vi "Master Configure Clock.vi"(8 "error in":errorcluster, 10 "Clock Source":T2(ring), 11 "Master Ref":T1) -> (0 "error out":errorcluster, 2 "Configuration Error":bool, 3 "Master Ref":T1)   [LabVIEW 2015]
doc: "This VI configures the clock source for the NI 5782. For execution steps, refer to the comments on the block diagram."
uses:
  Controls/FpgaMasterRef Typedef.ctl
  <vilib>/Utility/error.llb/Error Cluster From Error Code.vi
  <vilib>/rvi/errors/niLvFpgaAdjustHostInterfaceError.vi
  <vilib>/rvi/interface/nirviReadWriteControl/nirviReadWriteControl.xnode
  FPGA Bitfiles/LidarMasterV5.2.1.lvbitx
  NiFpgaLv.dll
panel:
  out "PLL Locked 2":bool
  out "ref":i32
  out "PLL Locked":bool
  # "This VI configures the clock source for the NI 5771. For execution steps, refer to the comments on the block diagram."
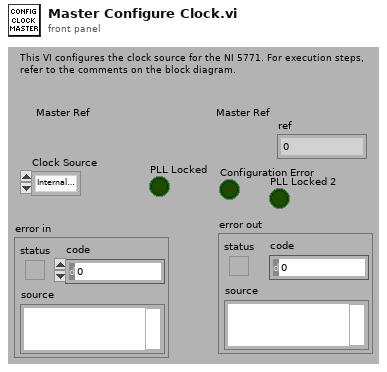
[diagram p1: front panel]
types:
  T1 = typedef "FpgaMasterRef Typedef.ctl" = refnum<k20>
  T2 = enum8{"Internal Clock PLL Off", "Internal Clock PLL On (CLK IN)", "External Clock (CLK IN)", "Internal Clock PLL On (IoModSyncClock)", "Extrernal Clock (IoModSyncClk)"}
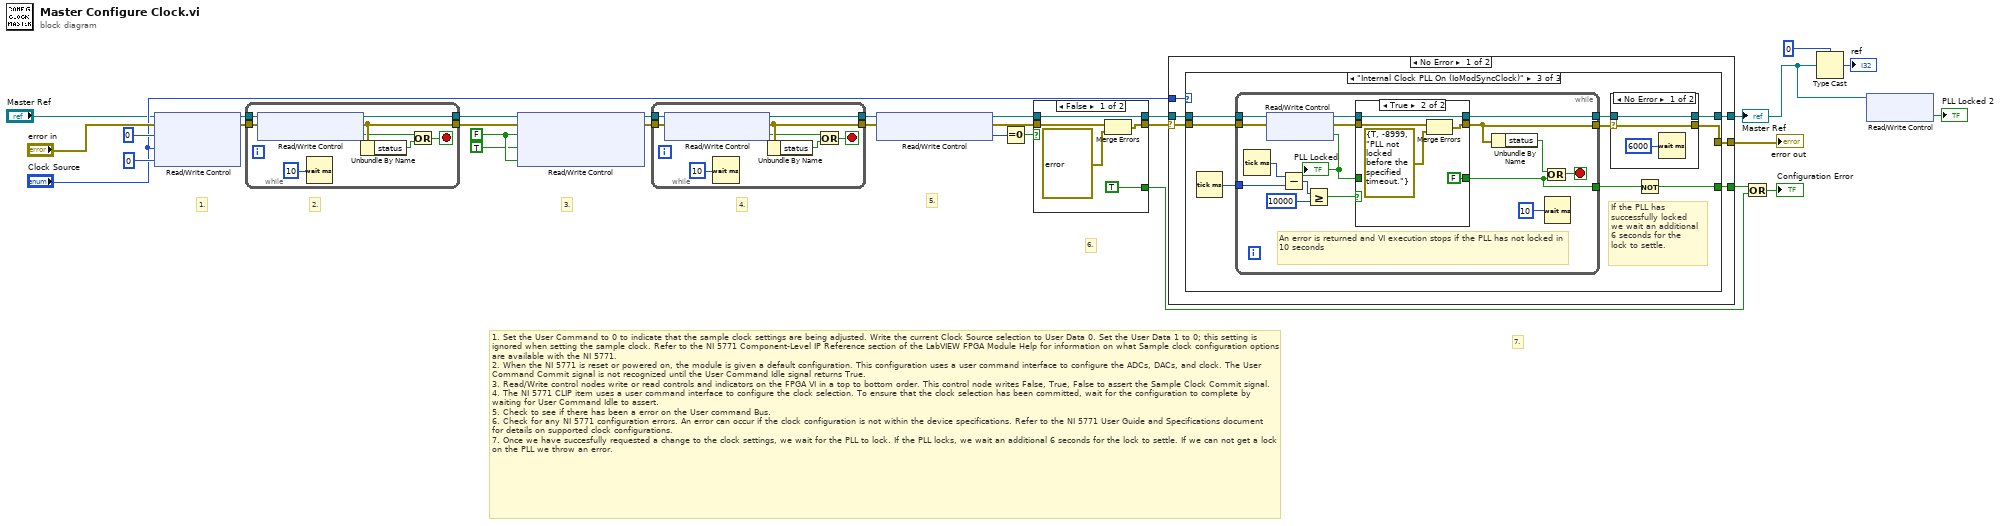
[diagram p0: block diagram]
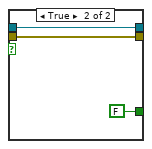
[diagram p2: hidden frame]
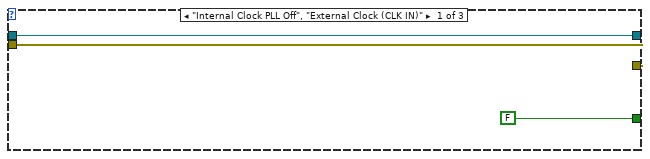
[diagram p3: hidden frame]
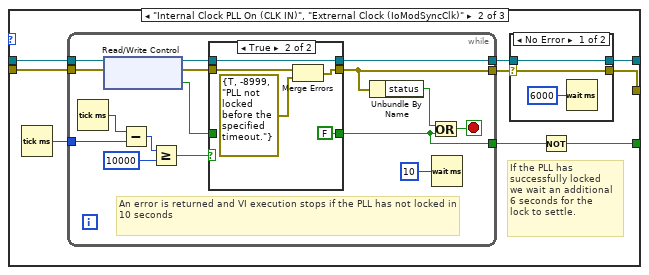
[diagram p4: hidden frame]
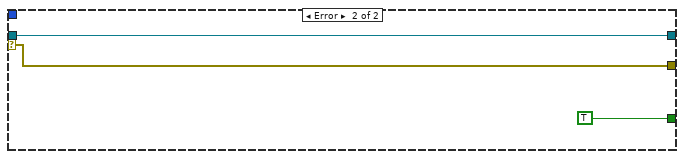
[diagram p9: hidden frame]
diagram:
  w24 = FALSE ("Sample Clock Commit")
  # "6."
  # "5."
  # "7."
  # "1. Set the User Command to 0 to indicate that the sample clock settings are being adjusted. Write the current Clock Source selection to User Data 0. Set the User Data 1 to 0; this setting is ignored when setting the sample clock. Refer to the NI 5771 Component-Level IP Reference section of the LabVIEW FPGA Module Help for information on what Sample clock configuration options are available with the NI 5771.\n2. When the NI 5771 is reset or powered on, the module is given a default configuration. This configuration uses a user command interface to configure the ADCs, DACs, and clock. The User Command Commit signal is not recognized until the User Command Idle signal returns True.\n3. Read/Write control nodes write or read controls and indicators on the FPGA VI in a top to bottom order. This control node writes False, True, False to assert the Sample Clock Commit signal.\n4. The NI 5771 CLIP item uses a user command interface to configure the clock selection. To ensure that the clock selection has been committed, wait for the configuration to complete by waiting for User Command Idle to assert.\n5. Check to see if there has been a error on the User command Bus. \n6. Check for any NI 5771 configuration errors. An error can occur if the clock configuration is not within the device specifications. Refer to the NI 5771 User Guide and Specifications document for details on supported clock configurations.\n7. Once we have succesfully requested a change to the clock settings, we wait for the PLL to lock. If the PLL locks, we wait an additional 6 seconds for the lock to settle. If we can not get a lock on the PLL we throw an error."
  # "4."
  # "3."
  # "2."
  # "1."
  n1 = xnode "Read/Write Control"("FPGA VI Reference In"="Master Ref", "error in"="error in", "User Command"=u8 0, "User Data 0"="Clock Source", "User Data 1"=u8 0) -> ("FPGA VI Reference Out"=w28:T1, "error out"=w27:errorcluster)
  n2 = while {
    tunnel: w28 -> [w33]
    tunnel: w27 -> [w34]
    tunnel: [w31] -> w25
    tunnel: [w32] -> w26
    stop <- w35 stop-if-true
    n3 = xnode "Read/Write Control"("FPGA VI Reference In"=w33, "error in"=w34) -> ("FPGA VI Reference Out"=w32:T1, "error out"=w31:errorcluster, "User Command Idle"=w30:bool)
    n4 = Wait (ms)(milliseconds to wait=u32 10) -> ()  [unwired: 1 out]
    n5 = Unbundle By Name(w31) -> ("status"=w36:bool)
    n6 = Or(x=w30, y=w36) -> (x .or. y?=w35:bool)
  }
  n7 = xnode "Read/Write Control"("FPGA VI Reference In"=w26, "error in"=w25, "User Command Commit"=w24, "User Command Commit"=TRUE ("Sample Clock Commit"), "User Command Commit"=w24) -> ("FPGA VI Reference Out"=w22:T1, "error out"=w21:errorcluster)
  n8 = while {
    tunnel: w22 -> [w41]
    tunnel: w21 -> [w42]
    tunnel: [w39] -> w20
    tunnel: [w40] -> w19
    stop <- w43 stop-if-true
    n9 = xnode "Read/Write Control"("FPGA VI Reference In"=w41, "error in"=w42) -> ("FPGA VI Reference Out"=w40:T1, "error out"=w39:errorcluster, "User Command Idle"=w38:bool)
    n10 = Wait (ms)(milliseconds to wait=u32 10) -> ()  [unwired: 1 out]
    n11 = Unbundle By Name(w39) -> ("status"=w44:bool)
    n12 = Or(x=w38, y=w44) -> (x .or. y?=w43:bool)
  }
  n13 = xnode "Read/Write Control"("FPGA VI Reference In"=w19, "error in"=w20) -> ("FPGA VI Reference Out"=w7:T1, "error out"=w9:errorcluster, "User Command Status"=w8:u8)
  n14 = Equal To 0?(x=w8) -> (x = 0?=w6:bool)
  n15 = case shown="False" w6 {
    tunnel: [w50 w53] -> w15
    tunnel: w9 -> [w49 w53]
    tunnel: [TRUE ("Configured?") FALSE ("Configured?")] -> w10
    tunnel: w7 -> [w46 w51]
    tunnel: [w46 w51] -> w13
    frame False {
      n16 = Merge Errors(w49, errorcluster {"status"=TRUE, "code"=-8998, "source"="IO Module clock not configured correctly. Please ensure that the desired clock meets the required specifications."} ("error in")) -> (w50:errorcluster)
    }
    frame True {
    }
  }
  n17 = case shown="No Error" w15 {
    selector: w15 -> [w57 w140]
    tunnel: "Clock Source" -> [w59 _]
    tunnel: w13 -> [w58 w141]
    tunnel: [w56 w140] -> w14
    tunnel: [w55 w141] -> w2
    tunnel: [w54 TRUE ("Configured?")] -> w12
    frame No Error {
      n18 = case shown="\"Internal Clock PLL On (IoModSyncClock)\"" w59 {
        tunnel: w58 -> [w61 w70 w108]
        tunnel: w57 -> [w62 w69 w107]
        tunnel: [w62 w66 w104] -> w56
        tunnel: [w61 w67 w105] -> w55
        tunnel: [FALSE ("Configured?") w63 w101] -> w54
        frame "Internal Clock PLL Off", "External Clock (CLK IN)" {
        }
        frame "Internal Clock PLL On (CLK IN)", "Extrernal Clock (IoModSyncClk)" {
          # "If the PLL has \nsuccessfully locked \nwe wait an additional\n6 seconds for the \nlock to settle."
          n19 = Tick Count (ms)() -> (millisecond timer value=w71:u32)
          n20 = while {
            tunnel: [w90] -> w68
            tunnel: w70 -> [w87]
            tunnel: w71 -> [w83]
            tunnel: w69 -> [w81]
            tunnel: [w78] -> w65
            tunnel: [w77] -> w64
            stop <- w88 stop-if-true
            # "An error is returned and VI execution stops if the PLL has not locked in 10 seconds"
            n21 = Tick Count (ms)() -> (millisecond timer value=w84:u32)
            n22 = xnode "Read/Write Control"("FPGA VI Reference In"=w87, "error in"=w81) -> ("FPGA VI Reference Out"=w79:T1, "error out"=w85:errorcluster, "PLL Locked"=w86:bool)
            n23 = Subtract(x=w84, y=w83) -> (x-y=w82:u32)
            n24 = Greater Or Equal?(x=w82, y=u32 10000) -> (x >= y?=w91:bool)
            n25 = case shown="True" w91 {
              tunnel: [w95 FALSE ("Configured?")] -> w77
              tunnel: w86 -> [w95 _]
              tunnel: [w94 w99] -> w90
              tunnel: w85 -> [w94 w97]
              tunnel: w79 -> [w93 w96]
              tunnel: [w93 w96] -> w78
              frame False {
              }
              frame True {
                n26 = Merge Errors(w97, errorcluster {"status"=TRUE, "code"=-8999, "source"="PLL not locked before the specified timeout."} ("error in")) -> (w99:errorcluster)
              }
            }
            n27 = Unbundle By Name(w90) -> ("status"=w89:bool)
            n28 = Or(x=w89, y=w77) -> (x .or. y?=w88:bool)
            n29 = Wait (ms)(milliseconds to wait=u32 10) -> ()  [unwired: 1 out]
          }
          n30 = case shown="No Error" w68 {
            selector: w68 -> [w72 w76]
            tunnel: w65 -> [w73 w75]
            tunnel: [w73 w75] -> w67
            tunnel: [w72 w76] -> w66
            frame No Error {
              n31 = Wait (ms)(milliseconds to wait=u32 6000) -> ()  [unwired: 1 out]
            }
            frame Error {
            }
          }
          n32 = Not(x=w64) -> (.not. x?=w63:bool)
        }
        frame "Internal Clock PLL On (IoModSyncClock)" {
          # "If the PLL has \nsuccessfully locked \nwe wait an additional\n6 seconds for the \nlock to settle."
          n33 = Tick Count (ms)() -> (millisecond timer value=w109:u32)
          n34 = while {
            tunnel: [w128] -> w106
            tunnel: w108 -> [w125]
            tunnel: w109 -> [w122]
            tunnel: w107 -> [w120]
            tunnel: [w117] -> w103
            tunnel: [w116] -> w102
            stop <- w126 stop-if-true
            # "An error is returned and VI execution stops if the PLL has not locked in 10 seconds"
            n35 = Tick Count (ms)() -> (millisecond timer value=w123:u32)
            n36 = xnode "Read/Write Control"("FPGA VI Reference In"=w125, "error in"=w120) -> ("FPGA VI Reference Out"=w118:T1, "error out"=w124:errorcluster, "PLL Locked"=w115:bool)
            "PLL Locked" <- w115
            n37 = Subtract(x=w123, y=w122) -> (x-y=w121:u32)
            n38 = Greater Or Equal?(x=w121, y=u32 10000) -> (x >= y?=w129:bool)
            n39 = case shown="True" w129 {
              tunnel: [w133 FALSE ("Configured?")] -> w116
              tunnel: w115 -> [w133 _]
              tunnel: [w132 w137] -> w128
              tunnel: w124 -> [w132 w135]
              tunnel: w118 -> [w131 w134]
              tunnel: [w131 w134] -> w117
              frame False {
              }
              frame True {
                n40 = Merge Errors(w135, errorcluster {"status"=TRUE, "code"=-8999, "source"="PLL not locked before the specified timeout."} ("error in")) -> (w137:errorcluster)
              }
            }
            n41 = Unbundle By Name(w128) -> ("status"=w127:bool)
            n42 = Or(x=w127, y=w116) -> (x .or. y?=w126:bool)
            n43 = Wait (ms)(milliseconds to wait=u32 10) -> ()  [unwired: 1 out]
          }
          n44 = case shown="No Error" w106 {
            selector: w106 -> [w110 w114]
            tunnel: w103 -> [w111 w113]
            tunnel: [w111 w113] -> w105
            tunnel: [w110 w114] -> w104
            frame No Error {
              n45 = Wait (ms)(milliseconds to wait=u32 6000) -> ()  [unwired: 1 out]
            }
            frame Error {
            }
          }
          n46 = Not(x=w102) -> (.not. x?=w101:bool)
        }
      }
    }
    frame Error {
    }
  }
  "error out" <- w14
  "Master Ref" <- w2
  n47 = Or(x=w12, y=w10) -> (x .or. y?=→"Configuration Error":bool)
  n48 = Type Cast(type=0, x=w2) -> (*(type *) &x=→"ref":i32)
  n49 = xnode "Read/Write Control"("FPGA VI Reference In"=w2) -> ("PLL Locked"=→"PLL Locked 2":bool)  [unwired: 1 in, 2 out]
